vi "TDD Spec String.vi"(11 "Spec String":string) -> (0 "Mating LowerSpec":dbl, 1 "Cable UpperSpec":dbl, 2 "Mating UpperSpec":dbl, 3 "CableArea":dbl, 4 "Cable LowerSpec":dbl, 5 "MatingArea":dbl)   [LabVIEW 2011]
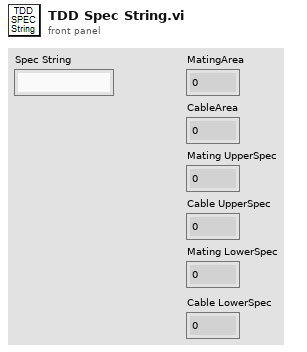
[diagram p1: front panel]
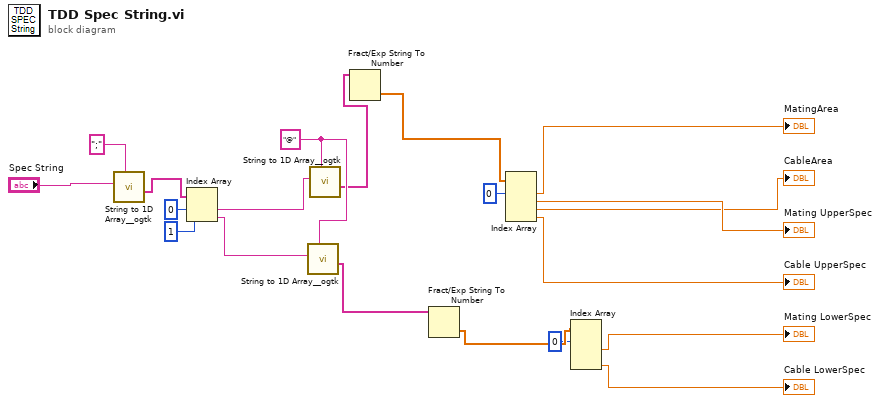
[diagram p0: block diagram]
diagram:
  w14 = "@" ("delimiter (Tab)")
  n1 = call <userlib>:"String to 1D Array__ogtk.vi"("delimiter (Tab)"=";", "string"="Spec String") -> ("Array of Strings"=w19:string[])  [unwired: 9 in]
  n2 = Index Array(array=w19, index #1=0 ("索引"), index #2=1 ("索引")) -> (element #1=w16:string, element #2=w15:string)
  n3 = call <userlib>:"String to 1D Array__ogtk.vi"("delimiter (Tab)"=w14, "string"=w15) -> ("Array of Strings"=w6:string[])  [unwired: 9 in]
  n4 = call <userlib>:"String to 1D Array__ogtk.vi"("delimiter (Tab)"=w14, "string"=w16) -> ("Array of Strings"=w12:string[])  [unwired: 9 in]
  n5 = Fract/Exp String To Number(string=w12) -> (number=w11:dbl[])  [unwired: 3 in, 1 out]
  n6 = Fract/Exp String To Number(string=w6) -> (number=w5:dbl[])  [unwired: 3 in, 1 out]
  n7 = Index Array(array=w11, index #1=0 ("索引")) -> (element #1=→"MatingArea":dbl, element #2=→"Mating UpperSpec":dbl, element #3=→"CableArea":dbl, element #4=→"Cable UpperSpec":dbl)  [unwired: 3 in]
  n8 = Index Array(array=w5, index #1=0 ("索引")) -> (element #2=→"Mating LowerSpec":dbl, element #4=→"Cable LowerSpec":dbl)  [unwired: 3 in, 2 out]
